vi "GetPPMSStatus.vi"() -> ()   [LabVIEW 2013]
uses:
  C:/QdLabview/QDInstrument.dll
panel:
  out "Field Status":dbl
  out "Field":dbl
  out "Temp Status":dbl
  out "Temp":dbl
  in  "Instrument\nType 2":i32(ring) items=["PPMS", "VersaLab", "DynaCool", "SVSM"]
  in  "Remote 2":bool
  in  "IP Address 2":string="127.0.0.1"
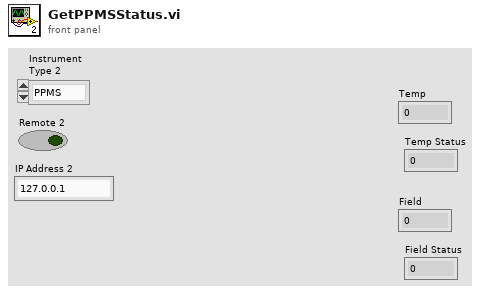
[diagram p1: front panel]
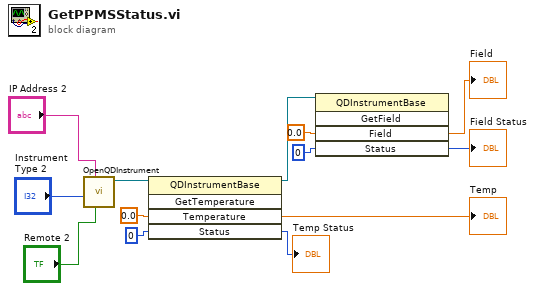
[diagram p0: block diagram]
diagram:
  n1 = call "OpenQDInstrument.vi"("Remote"="Remote 2", "IP Address"="IP Address 2", "Instrument Type"="Instrument\nType 2") -> ("Instrument Ref"=w8:refnum<k24>)  [unwired: 5 in, 1 out]
  n2 = invoke class="QDInstrumentBase" method="GetTemperature"(reference=w8, "Temperature"=0.0, "Status"=0) -> (reference out=w1:refnum<k24>, "Temperature"=→"Temp":dbl, "Status"=→"Temp Status":i32)  [unwired: 2 in, 2 out]
  n3 = invoke class="QDInstrumentBase" method="GetField"(reference=w1, "Field"=0.0 ("Temperature"), "Status"=0) -> ("Field"=→"Field":dbl, "Status"=→"Field Status":i32)  [unwired: 2 in, 3 out]
